vi "Get Created.vi"(11 "Addresses Strategy in":refnum<class "Addresses Strategy.lvclass">) -> (2 "Created":T1)   [LabVIEW 2021, in "jettl.lvlib" / "Addresses Strategy.lvlib" / "Addresses Strategy.lvclass"]
uses:
  Addresses Strategy.lvclass
  Created.ctl
  Msg/Msg.lvclass
  Addresses Strategy.lvlib
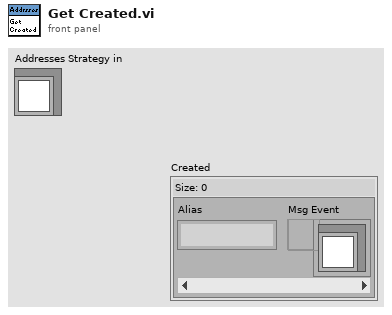
[diagram p1: front panel]
types:
  T1 = typedef "jettl.lvlib/Addresses Strategy.lvlib/Created.ctl" = map{string, refnum<user-event>}
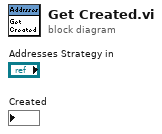
[diagram p0: block diagram]
diagram:
